vi "PH_PP_CurrentMeas.calc Status.vi"(0 "i ref in":refnum<vi>, 5 "error in (no error)":errorcluster) -> (14 "i ref out":refnum<vi>, 19 "error out":errorcluster)   [LabVIEW 2014, in "PH_PP_CurrentMeas.lvlib"]
uses:
  PH_PP_CurrentMeas.lvlib
  PH_Basics/PH_StatusHandler/PH_StatusHandler.Status.ctl
  PH_Basics/PH_StatusHandler/PH_StatusHandler.lvlib
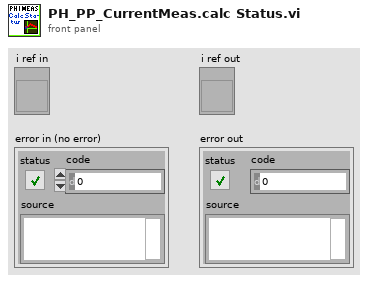
[diagram p1: front panel]
types:
  T1 = typedef "PH_StatusHandler.lvlib/PH_StatusHandler.Status.ctl" = i16
  T2 = typedef "PH_PP_CurrentMeas.lvlib/PH_PP_CurrentMeas.i attribute.ctl" = cluster{"Status":cluster{"GUI Ref Hardware Feedback":refnum<vi>, "Tab Control":refnum<vi>}, "PU 1":cluster{"Instance":string, "Status":T1, "Ref Status ":refnum<vi>, "Data":waveform(dbl)[], "Ref Data":refnum<vi>}, "PU 2":cluster{"Instance":string, "Status":T1, "Ref Status ":refnum<vi>, "Data":waveform(dbl)[], "Ref Data":refnum<vi>}, "PU 3":cluster{"Instance":string, "Status":T1, "Ref Status ":refnum<vi>, "Data":waveform(dbl)[], "Ref Data":refnum<vi>}, "PU 4":cluster{"Instance":string, "Status":T1, "Ref Status ":refnum<vi>, "Data":waveform(dbl)[], "Ref Data":refnum<vi>}, "PU 5":cluster{"Instance":string, "Status":T1, "Ref Status ":refnum<vi>, "Data":waveform(dbl)[], "Ref Data":refnum<vi>}, "FR":cluster{"Instance":string, "Status":T1, "Ref Status ":refnum<vi>, "Data":waveform(dbl)[], "Ref Data":refnum<vi>}, "PA - 19mm 1":cluster{"Instance":string, "Status":T1, "Ref Status ":refnum<vi>}, "PA - 19mm 2":cluster{"Instance":string, "Status":T1, "Ref Status ":refnum<vi>, "no link":bool}, "PA - 45mm":cluster{"Instance":string, "Status":T1, "Ref Status ":refnum<vi>, "no link":bool}, "PA Data":cluster{"Data":waveform(dbl)[], "Ref":refnum<vi>}, "Sequencer":cluster{"Instance":string, "SM State Ref":refnum<vi>}, "Tasks":cluster{"Port":u16, "connection ID":refnum<k5>, "Status":T1, "Ref":refnum<vi>, "Ref Bar":refnum<vi>, "Feedback":cluster{"Received Data Sets":T3[], "Driver Error":errorcluster, "Connection not established":bool, "Error unpacking the data":bool, "No Task defined":bool, "Not triggered yet":bool}, "Data":waveform(dbl)[], "Ref Teststart Task":refnum<vi>}[], "in use":cluster{"MA DP":bool, "FR and PA":bool}, "DAQ Server":string}
  T3 = typedef "PH_PP_CurrentMeas.lvlib/PH_PP_CurrentMeas.CommandCluster.ctl" = cluster{"Command":string, "Data":string, "error out":errorcluster}
  T4 = cluster{"Port":u16, "connection ID":refnum<k5>, "Status":T1, "Ref":refnum<vi>, "Ref Bar":refnum<vi>, "Feedback":cluster{"Received Data Sets":T3[], "Driver Error":errorcluster, "Connection not established":bool, "Error unpacking the data":bool, "No Task defined":bool, "Not triggered yet":bool}, "Data":waveform(dbl)[], "Ref Teststart Task":refnum<vi>}[]
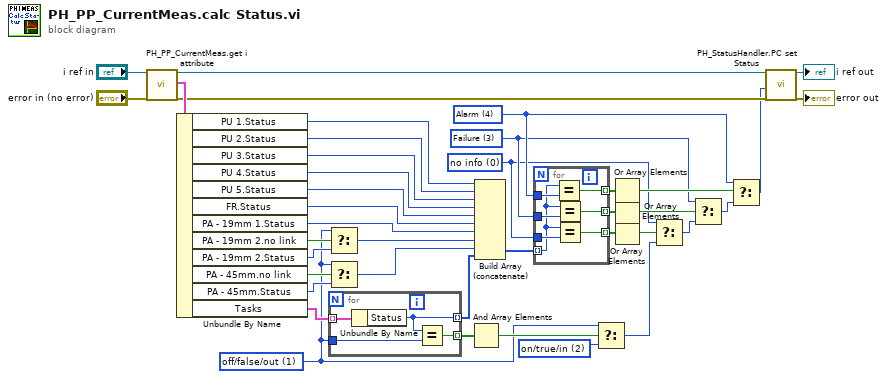
[diagram p0: block diagram]
diagram:
  w13 = T1 2 items=["no info", "off/false/out", "on/true/in", "Failure", "Alarm", "Status 1", "Status 2", "Status 3"] ("f")
  w4 = T1 1 items=["no info", "off/false/out", "on/true/in", "Failure", "Alarm", "Status 1", "Status 2", "Status 3"] ("y")
  w25 = T1 4 items=["no info", "off/false/out", "on/true/in", "Failure", "Alarm", "Status 1", "Status 2", "Status 3"] ("y")
  w21 = T1 3 items=["no info", "off/false/out", "on/true/in", "Failure", "Alarm", "Status 1", "Status 2", "Status 3"] ("y")
  w18 = T1 0 items=["no info", "off/false/out", "on/true/in", "Failure", "Alarm", "Status 1", "Status 2", "Status 3"] ("y")
  n1 = call "PH_PP_CurrentMeas.get i attribute.vi"("i ref in"="i ref in", "error in (no error)"="error in (no error)") -> ("i ref out"=w2:refnum<vi>, "i attribute"=w38:T2, "error out"=w12:errorcluster)  [unwired: 15 in]
  n2 = Unbundle By Name(w38) -> ("PU 1.Status"=w37:T1, "PU 2.Status"=w36:T1, "PU 3.Status"=w35:T1, "PU 4.Status"=w34:T1, "PU 5.Status"=w33:T1, "FR.Status"=w32:T1, "PA - 19mm 1.Status"=w31:T1, "PA - 19mm 2.no link"=w10:bool, "PA - 19mm 2.Status"=w9:T1, "PA - 45mm.no link"=w7:bool, "PA - 45mm.Status"=w6:T1, "Tasks"=w30:T4)
  n3 = Select(t=w4, s=w10, f=w9) -> (s? t:f=w8:T1)
  n4 = Select(t=w4, s=w7, f=w6) -> (s? t:f=w5:T1)
  n5 = for {
    tunnel: w30 -> [w44] mode=indexing
    tunnel: [w43] -> w29 mode=indexing
    tunnel: w4 -> [w42]
    tunnel: [w41] -> w15 mode=indexing
    n6 = Unbundle By Name(w44) -> ("Status"=w43:T1)
    n7 = Equal?(x=w43, y=w42) -> (x = y?=w41:bool)
  }
  n8 = And Array Elements(Boolean array=w15) -> (logical AND=w14:bool)
  n9 = Build Array (concatenate)(w37, w36, w35, w34, w33, w32, w31, w8, w5, w29) -> (w28:T1[])
  n10 = for {
    tunnel: w28 -> [w45] mode=indexing
    tunnel: w18 -> [w51]
    tunnel: w25 -> [w50]
    tunnel: w21 -> [w49]
    tunnel: [w48] -> w27 mode=indexing
    tunnel: [w47] -> w24 mode=indexing
    tunnel: [w46] -> w20 mode=indexing
    n11 = Equal?(x=w45, y=w50) -> (x = y?=w48:bool)
    n12 = Equal?(x=w45, y=w49) -> (x = y?=w47:bool)
    n13 = Equal?(x=w45, y=w51) -> (x = y?=w46:bool)
  }
  n14 = Select(t=w4, s=w14, f=w13) -> (s? t:f=w16:T1)
  n15 = Or Array Elements(Boolean array=w27) -> (logical OR=w26:bool)
  n16 = Or Array Elements(Boolean array=w24) -> (logical OR=w23:bool)
  n17 = Or Array Elements(Boolean array=w20) -> (logical OR=w19:bool)
  n18 = Select(t=w18, s=w19, f=w16) -> (s? t:f=w17:T1)
  n19 = Select(t=w21, s=w23, f=w17) -> (s? t:f=w22:T1)
  n20 = Select(t=w25, s=w26, f=w22) -> (s? t:f=w11:T1)
  n21 = call "PH_StatusHandler.PC set Status.vi"("i ref in"=w2, "Status"=w11, "error in (no error)"=w12) -> ("i ref out"=→"i ref out":refnum<vi>, "error out"=→"error out":errorcluster)  [unwired: 15 in]
